vi "RSD Responce Bytes Count.vi"(1 "Count Number":u8) -> (0 "Bytes Count":u32)   [LabVIEW 2016, in "Samwontech TEMP2xxx.lvlib"]
uses:
  <instrlib>/Samwontech TEMP2xxx/Samwontech TEMP2xxx.lvlib
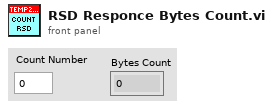
[diagram p1: front panel]
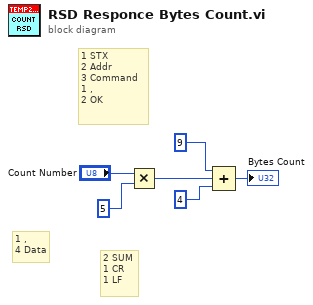
[diagram p0: block diagram]
diagram:
  # "1 ,\n4 Data"
  # "2 SUM\n1 CR\n1 LF"
  # "1 STX\n2 Addr\n3 Command\n1 ,\n2 OK"
  n1 = Multiply(x="Count Number", y=u8 5) -> (x*y=w4:u8)
  n2 = Compound Arithmetic op=unknown(u32 9, w4, u32 4 ("value")) -> (→"Bytes Count":u32)
